vi "laserInitGen.vi"(7 "647prop":T2, 8 "error in (no error)":errorcluster, 9 "553prop":T2, 10 "488prop":T2, 11 "Laser":T1={"488 nm"=0.0, "488on"=FALSE, "488mod"=FALSE, "553 nm"=0.0, "553on"=FALSE, "553mod"=FALSE, "647 nm"=0.0, "647on"=FALSE, "647mod"=FALSE, "488key"=FALSE, "488inter"=FALSE, "488err"=FALSE, "488mode"="conPow", "553key"=FALSE, "553inter"=FALSE, "553err"=FALSE, "553mode"="conPow", "647key"=FALSE, "647inter"=FALSE, "647err"=FALSE, "647mode"="conPow", "laser available"=TRUE, "488unit"="", "553unit"="", "647unit"=""} {"647 nm" format="%.2g"; "553 nm" format="%.2g"; "488 nm" format="%1.2g"}) -> (0 "error out":errorcluster, 1 "LaserPropOut488":T2, 2 "LaserPropOut553":T2, 3 "Laser 2":T1={"488 nm"=0.0, "488on"=FALSE, "488mod"=FALSE, "553 nm"=0.0, "553on"=FALSE, "553mod"=FALSE, "647 nm"=0.0, "647on"=FALSE, "647mod"=FALSE, "488key"=FALSE, "488inter"=FALSE, "488err"=FALSE, "488mode"="conPow", "553key"=FALSE, "553inter"=FALSE, "553err"=FALSE, "553mode"="conPow", "647key"=FALSE, "647inter"=FALSE, "647err"=FALSE, "647mode"="conPow", "laser available"=TRUE, "488unit"="", "553unit"="", "647unit"=""} {"647 nm" format="%.2g"; "553 nm" format="%.2g"; "488 nm" format="%1.2g"}, 5 "LaserPropOut647":T2)   [LabVIEW 2021]
panel:
  # "ON"
  # "Mode"
  # "Error-kei"
  # "ON"
  # "Mode"
  # "Error-kei"
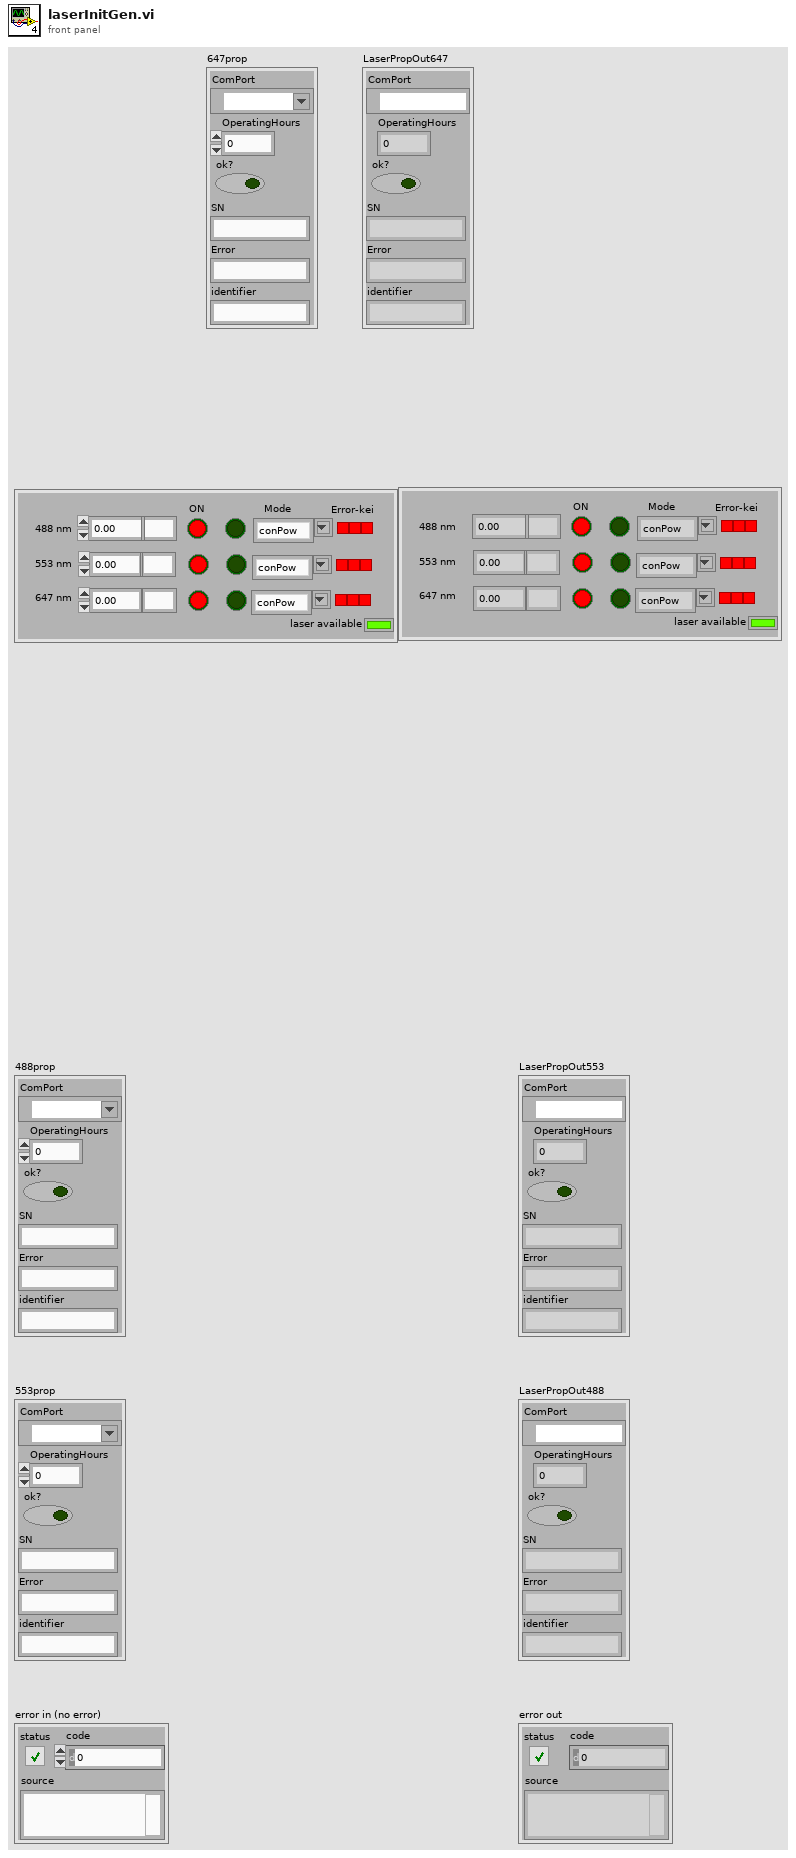
[diagram p1: front panel]
types:
  T1 = cluster{"488 nm":dbl, "488on":bool, "488mod":bool, "553 nm":dbl, "553on":bool, "553mod":bool, "647 nm":dbl, "647on":bool, "647mod":bool, "488key":bool, "488inter":bool, "488err":bool, "488mode":string, "553key":bool, "553inter":bool, "553err":bool, "553mode":string, "647key":bool, "647inter":bool, "647err":bool, "647mode":string, "laser available":bool, "488unit":string, "553unit":string, "647unit":string}
  T2 = cluster{"ComPort":refnum<visa-resource-name>, "OperatingHours":dbl, "ok?":bool, "SN":string, "Error":string, "identifier":string}
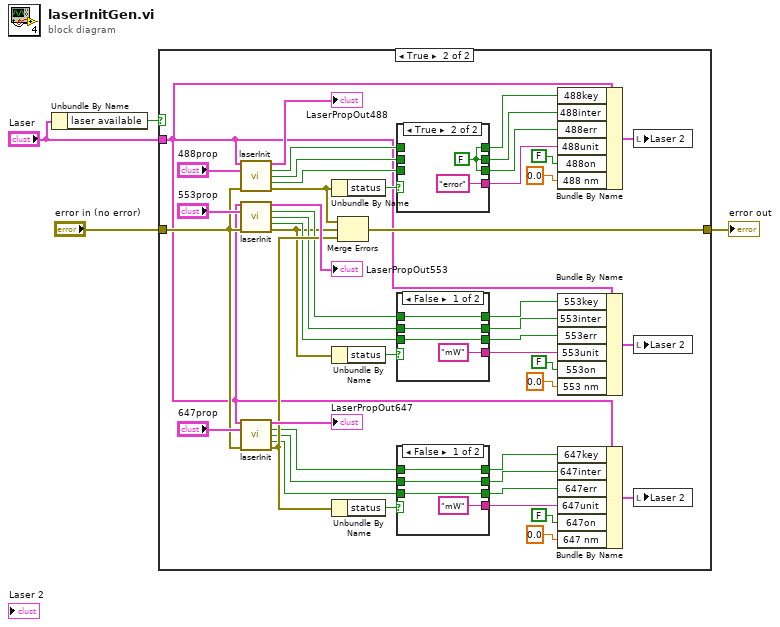
[diagram p0: block diagram]
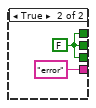
[diagram p3: hidden frame]
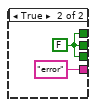
[diagram p4: hidden frame]
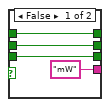
[diagram p5: hidden frame]
diagram:
  n1 = Unbundle By Name("Laser") -> ("laser available"=w2:bool)
  n2 = case shown="True" w2 {
    tunnel: [w5 w43] -> w4
    tunnel: "error in (no error)" -> [w5 w44]
    tunnel: "Laser" -> [_ w15]
    frame False {
    }
    frame True {
      n3 = call "laserInit.vi"("Laser"=w15, "LaserPropIn"="488prop", "error in (no error)"=w44) -> ("LaserPropOut"=→"LaserPropOut488":T2, "keySwitch"=w35:bool, "interLock"=w34:bool, "error"=w33:bool, "error out"=w42:errorcluster)  [unwired: 8 in]
      n4 = call "laserInit.vi"("Laser"=w15, "LaserPropIn"="553prop", "error in (no error)"=w44) -> ("LaserPropOut"=→"LaserPropOut553":T2, "keySwitch"=w14:bool, "interLock"=w13:bool, "error"=w12:bool, "error out"=w11:errorcluster)  [unwired: 8 in]
      n5 = call "laserInit.vi"("Laser"=w15, "LaserPropIn"="647prop", "error in (no error)"=w44) -> ("LaserPropOut"=→"LaserPropOut647":T2, "keySwitch"=w8:bool, "interLock"=w7:bool, "error"=w6:bool, "error out"=w41:errorcluster)  [unwired: 8 in]
      n6 = Unbundle By Name(w42) -> ("status"=w40:bool)
      n7 = Unbundle By Name(w11) -> ("status"=w10:bool)
      n8 = Unbundle By Name(w41) -> ("status"=w9:bool)
      n9 = Merge Errors(w42, w11, w41) -> (w43:errorcluster)
      n10 = case shown="True" w40 {
        tunnel: [w66 w68] -> w38
        tunnel: [w65 w68] -> w37
        tunnel: [w64 w68] -> w36
        tunnel: w35 -> [w66 _]
        tunnel: w34 -> [w65 _]
        tunnel: w33 -> [w64 _]
        tunnel: ["mW" "error"] -> w32
        frame False {
        }
        frame True {
          w68 = FALSE
        }
      }
      n11 = case shown="False" w10 {
        tunnel: [w60 w62] -> w24
        tunnel: [w59 w62] -> w25
        tunnel: [w58 w62] -> w26
        tunnel: w14 -> [w60 _]
        tunnel: w13 -> [w59 _]
        tunnel: w12 -> [w58 _]
        tunnel: ["mW" "error"] -> w27
        frame False {
        }
        frame True {
          w62 = FALSE
        }
      }
      n12 = case shown="False" w9 {
        tunnel: [w54 w56] -> w21
        tunnel: [w53 w56] -> w20
        tunnel: [w52 w56] -> w19
        tunnel: w8 -> [w54 _]
        tunnel: w7 -> [w53 _]
        tunnel: w6 -> [w52 _]
        tunnel: ["mW" "error"] -> w18
        frame False {
        }
        frame True {
          w56 = FALSE
        }
      }
      n13 = Bundle By Name(cluster=w15, "488key"=w38, "488inter"=w37, "488err"=w36, "488unit"=w32, "488on"=FALSE, "488 nm"=0.0) -> (w39:T1)
      n14 = Bundle By Name(cluster=w15, "553key"=w24, "553inter"=w25, "553err"=w26, "553unit"=w27, "553on"=FALSE, "553 nm"=0.0 ("488 nm")) -> (w23:T1)
      n15 = Bundle By Name(cluster=w15, "647key"=w21, "647inter"=w20, "647err"=w19, "647unit"=w18, "647on"=FALSE, "647 nm"=0.0 ("488 nm")) -> (w22:T1)
      n16 = local write "Laser 2"(w39) -> ()
      n17 = local write "Laser 2"(w23) -> ()
      n18 = local write "Laser 2"(w22) -> ()
    }
  }
  "error out" <- w4
